vi "SetOutputState.vi"(8 "error in (no error)":errorcluster, 10 "Output State":bool, 11 "Cooler in":refnum<class "Cooler.lvclass">) -> (0 "error out":errorcluster, 3 "Cooler out":refnum<class "Cooler.lvclass">)   [LabVIEW 2015, in "Cooler.lvlib" / "Cooler.lvclass"]
uses:
  Cooler.lvclass
  Cooler.lvclass/Cooler.ctl
  Cooler UI/Cooler UI with Events Messages/Message Update Pump/Message Update Pump.lvclass/Message Update Pump.ctl
  <vilib>/ActorFramework/Message Enqueuer/Message Enqueuer.lvclass/Message Enqueuer.ctl
  <vilib>/ActorFramework/Time-Delayed Send Message/Time-Delay Override Options.ctl
  Dual Controller/Dual Fan Messages/Message Power On/Message Power On.lvclass
  <vilib>/ActorFramework/Message Enqueuer/Enqueue.vi
  <vilib>/ActorFramework/Message Priority Queue/Priority Enqueue.vi
  Simulation/Simulation Data_Global.vi
  Cooler UI/Cooler UI with Events Messages/Message Update Pump/Message Update Pump.lvclass
  Dual Controller/Dual Fan Messages/Message Power Off/Message Power Off.lvclass
  Simulation/Simulation.lvlib
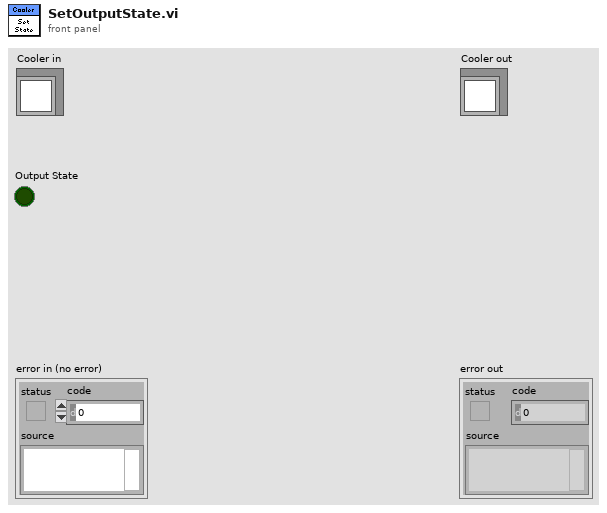
[diagram p1: front panel]
types:
  T1 = typedef "Time-Delay Override Options.ctl" = enum16{"Send next copy now", "Skip next scheduled copy", "Send next copy now and stop all further copies", "Stop all further copies"}
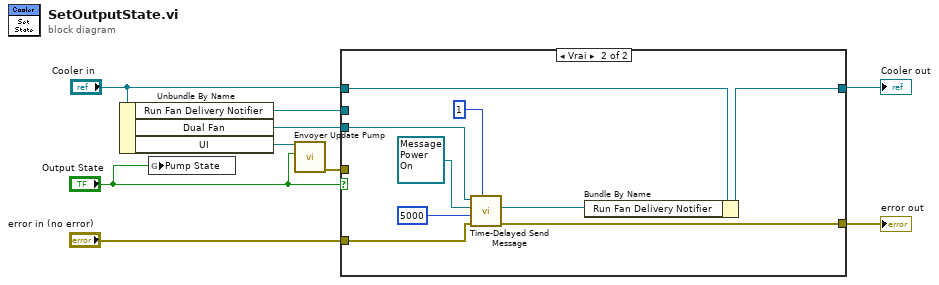
[diagram p0: block diagram]
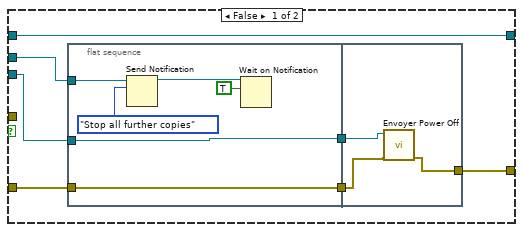
[diagram p2: hidden frame]
diagram:
  n1 = Unbundle By Name("Cooler in") -> ("Run Fan Delivery Notifier"=w7:refnum<notifier>, "Dual Fan"=w5:refnum<class "Message Enqueuer.lvclass">, "UI"=w3:refnum<class "Message Enqueuer.lvclass">)
  n2 = global write "Simulation Data_Global.vi" "Pump State"("Output State") -> ()
  n3 = call "Envoyer Update Pump.vi"("Pump State"="Output State", "Message Enqueuer"=w3) -> ("error out"=w1:errorcluster)  [unwired: 8 in, 1 out]
  n4 = case shown="Vrai" "Output State" {
    tunnel: "error in (no error)" -> [w14 w29]
    tunnel: "Cooler in" -> [w16 w34]
    tunnel: [w16 w33] -> w8
    tunnel: w7 -> [w13 _]
    tunnel: w5 -> [w11 w32]
    tunnel: [w10 w28] -> w4
    tunnel: w1 -> [_ _]
    frame False {
      n5 = flat-sequence {
        tunnel: w13 -> [w20]
        tunnel: [w22] -> w15
        tunnel: w14 -> [w22]
        tunnel: [w21] -> w12
        tunnel: w11 -> [w21]
        tunnel: w15 -> [w25]
        tunnel: w12 -> [w23]
        tunnel: [w24] -> w10
        frame #0 {
          n6 = Send Notification(notification=Time-Delay_Override_Options."Stop all further copies", notifier=w20) -> (notifier out=w18:refnum<notifier>)  [unwired: 1 in, 1 out]
          n7 = Wait on Notification(notifier=w18, ignore previous (F)=TRUE ("ignorer les précédents (F)")) -> ()  [unwired: 2 in, 4 out]
        }
        frame #1 {
          n8 = call "Envoyer Power Off.vi"("error in (no error)"=w25, "Message Enqueuer"=w23) -> ("error out"=w24:errorcluster)  [unwired: 8 in, 1 out]
        }
      }
    }
    frame True {
      n9 = call <vilib>:"Time-Delayed Send Message.vi"("# Copies (0 = infinite repeat)"=u32 1, "error in (no error)"=w29, "Milliseconds To Wait"=5000, "Message"=refnum<class "Message Power On.lvclass"> refnum ("Dual Fan.lvlib:Message Power On.lvclass"), "Message Enqueuer"=w32) -> ("error out"=w28:errorcluster, "Delivery Notifier"=w27:refnum<notifier>)  [unwired: 5 in]
      n10 = Bundle By Name(cluster=w34, "Run Fan Delivery Notifier"=w27) -> (w33:refnum<class "Cooler.lvclass">)
    }
  }
  "error out" <- w4
  "Cooler out" <- w8
